vi "Feader.vi"(11 "SHOOT Button":bool) -> (3 "Ready To Shoot?":bool)   [LabVIEW 2012]
uses:
  <vilib>/Rock Robotics/WPI/Solenoid/Deprecated/WPI_SolenoidSetBool.vi
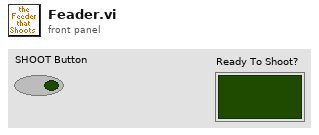
[diagram p1: front panel]
types:
  T1 = typedef "WPI_SolenoidDevRef.ctl" = cluster{"DevStatus":errorcluster, "Solenoid Module":T2, "Forward Solenoid Channel":T3, "Reverse Solenoid Channel":T3}
  T2 = typedef "FPGA_TypedefSolenoidModule.ctl" = enum16{"Solenoid Module 1", "Solenoid Module 2"}
  T3 = typedef "WPI_SolenoidChannel.ctl" = enum8{"Solenoid 1", "Solenoid 2", "Solenoid 3", "Solenoid 4", "Solenoid 5", "Solenoid 6", "Solenoid 7", "Solenoid 8", "Invalid"}
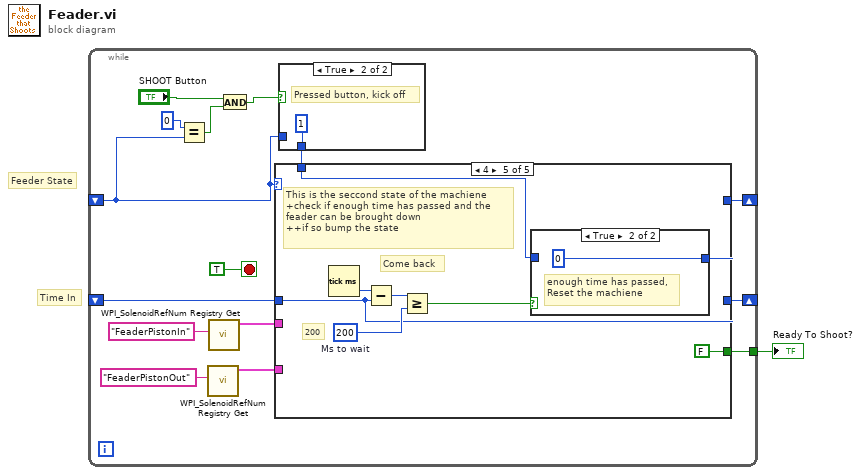
[diagram p0: block diagram]
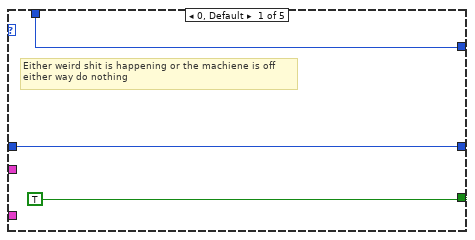
[diagram p2: hidden frame]
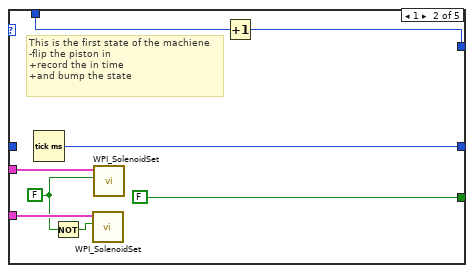
[diagram p3: hidden frame]
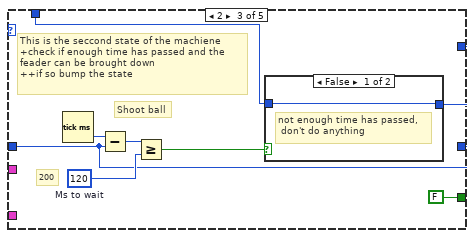
[diagram p4: hidden frame]
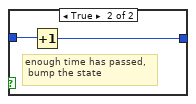
[diagram p5: hidden frame]
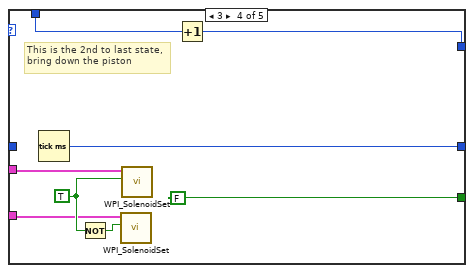
[diagram p6: hidden frame]
diagram:
  # "Feeder State"
  # "Time In"
  n1 = while {
    tunnel: [w14] -> w1
    shift-right: [w7] -> _
    shift-left: _ -> [w10]
    shift-right: [w8] -> _
    shift-left: _ -> [w2]
    stop <- TRUE stop-if-true
    n2 = Equal?(x=0, y=w2) -> (x = y?=w4:bool)
    n3 = call <vilib>:"WPI_SolenoidRefNum Registry Get.vi"("refnum name"="FeaderPistonOut") -> ("SolenoidDevRef"=w12:T1)  [unwired: 9 in, 1 out]
    n4 = call <vilib>:"WPI_SolenoidRefNum Registry Get.vi"("refnum name"="FeaderPistonIn") -> ("SolenoidDevRef"=w13:T1)  [unwired: 9 in, 1 out]
    n5 = And(x="SHOOT Button", y=w4) -> (x .and. y?=w3:bool)
    n6 = case shown="True" w3 {
      tunnel: [w57 1] -> w9
      tunnel: w2 -> [w57 _]
      frame False {
        # "Not pressed button"
      }
      frame True {
        # "Pressed button, kick off"
      }
    }
    n7 = case shown="4" w2 {
      tunnel: [TRUE FALSE FALSE FALSE FALSE] -> w14
      tunnel: w13 -> [_ w26 _ w44 _]
      tunnel: w12 -> [_ w25 _ w43 _]
      tunnel: w10 -> [w17 _ w28 _ w47]
      tunnel: w9 -> [w18 w21 w30 w40 w49]
      tunnel: [w18 w20 w29 w39 w48] -> w8
      tunnel: [w17 w22 w28 w41 w47] -> w7
      frame 0, Default {
        # "Either weird shit is happening or the machiene is off\neither way do nothing"
      }
      frame 1 {
        w23 = FALSE
        # "This is the first state of the machiene\n-flip the piston in\n+record the in time\n+and bump the state"
        n8 = Tick Count (ms)() -> (millisecond timer value=w22:u32)
        n9 = Not(x=w23) -> (.not. x?=w24:bool)
        n10 = call-poly <vilib>:"WPI_SolenoidSet.vi"("Value"=w24, "SolenoidDevRef"=w25) -> ()  [unwired: 8 in, 2 out]
        n11 = call-poly <vilib>:"WPI_SolenoidSet.vi"("Value"=w23, "SolenoidDevRef"=w26) -> ()  [unwired: 8 in, 2 out]
        n12 = Increment(x=w21) -> (x+1=w20:i32)
      }
      frame 2 {
        w33 = 120  # Ms to wait
        # "200"
        # "Shoot ball"
        # "This is the seccond state of the machiene\n+check if enough time has passed and the \nfeader can be brought down\n++if so bump the state"
        n13 = Tick Count (ms)() -> (millisecond timer value=w35:u32)
        n14 = Subtract(x=w35, y=w28) -> (x-y=w34:u32)
        n15 = Greater Or Equal?(x=w34, y=w33) -> (x >= y?=w31:bool)
        n16 = case shown="False" w31 {
          tunnel: w30 -> [w36 w37]
          tunnel: [w36 w38] -> w29
          frame False {
            # "not enough time has passed,\n don't do anything"
          }
          frame True {
            # "enough time has passed,\n bump the state"
            n17 = Increment(x=w37) -> (x+1=w38:i32)
          }
        }
      }
      frame 3 {
        w45 = TRUE
        # "This is the 2nd to last state,\nbring down the piston"
        n18 = Tick Count (ms)() -> (millisecond timer value=w41:u32)
        n19 = Not(x=w45) -> (.not. x?=w46:bool)
        n20 = call-poly <vilib>:"WPI_SolenoidSet.vi"("Value"=w46, "SolenoidDevRef"=w43) -> ()  [unwired: 8 in, 2 out]
        n21 = call-poly <vilib>:"WPI_SolenoidSet.vi"("Value"=w45, "SolenoidDevRef"=w44) -> ()  [unwired: 8 in, 2 out]
        n22 = Increment(x=w40) -> (x+1=w39:i32)
      }
      frame 4 {
        w52 = 200  # Ms to wait
        # "200"
        # "Come back"
        # "This is the seccond state of the machiene\n+check if enough time has passed and the \nfeader can be brought down\n++if so bump the state"
        n23 = Tick Count (ms)() -> (millisecond timer value=w54:u32)
        n24 = Subtract(x=w54, y=w47) -> (x-y=w53:u32)
        n25 = Greater Or Equal?(x=w53, y=w52) -> (x >= y?=w50:bool)
        n26 = case shown="True" w50 {
          tunnel: w49 -> [w55 _]
          tunnel: [w55 0] -> w48
          frame False {
            # "not enough time has passed,\n don't do anything"
          }
          frame True {
            # "enough time has passed,\nReset the machiene"
          }
        }
      }
    }
  }
  "Ready To Shoot?" <- w1
